vi "wfm_feature calc_repeat_range.vi"(8 "error in (no error)":errorcluster, 10 "limit data":cluster{"X":dbl, "Y":dbl}[](array[cluster]), 11 "wfm_feature in":refnum<class "wfm_feature.lvclass">) -> (0 "error out":errorcluster, 3 "wfm_feature out":refnum<class "wfm_feature.lvclass">)   [LabVIEW 2018, in "wfm_feature.lvclass"]
uses:
  wfm_feature.lvclass
  wfm_feature.lvclass/wfm_feature.ctl
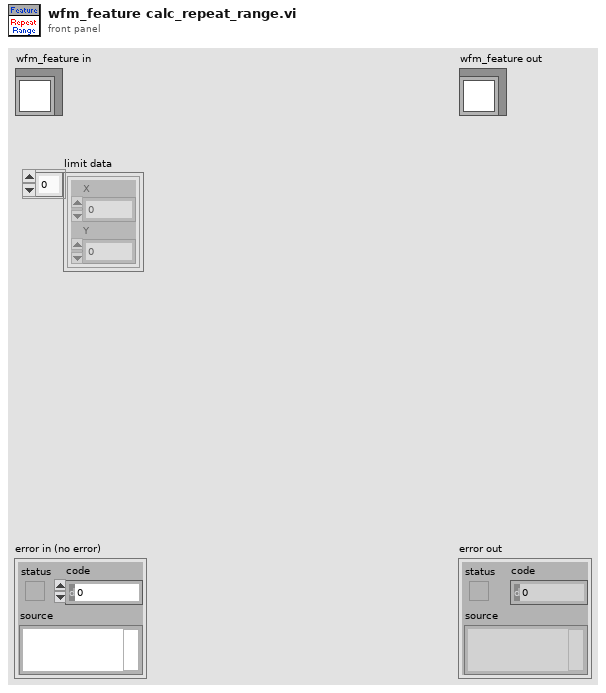
[diagram p1: front panel]
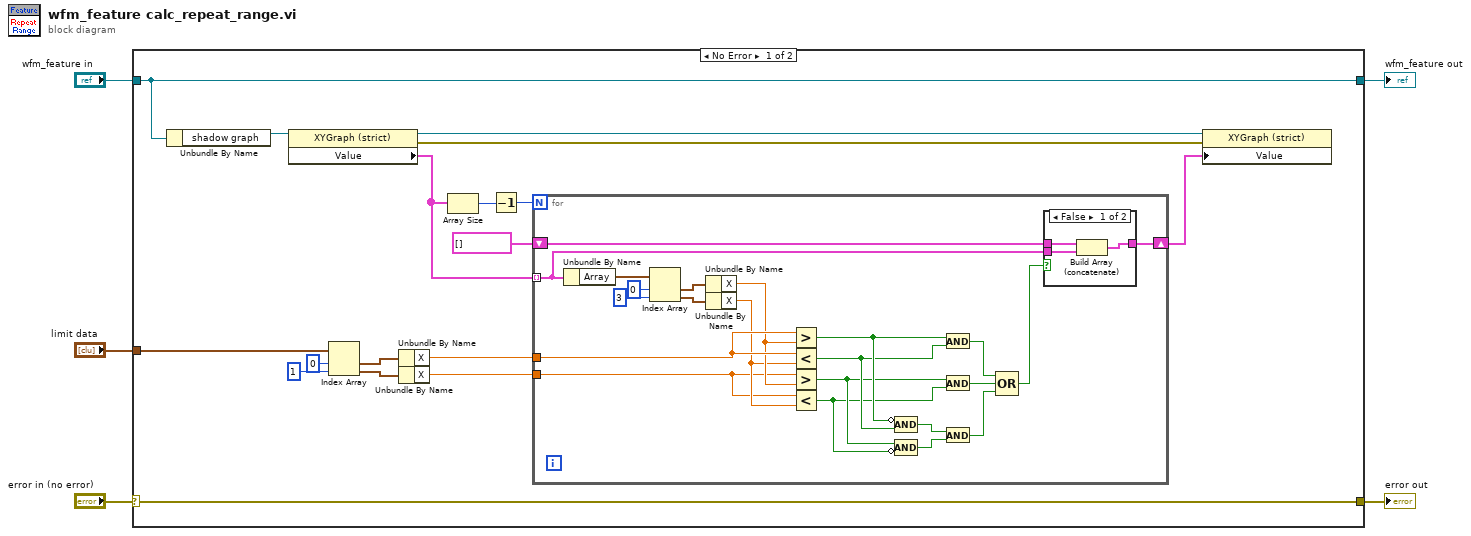
[diagram p0: block diagram]
diagram:
  n1 = case shown="No Error" "error in (no error)" {
    selector: "error in (no error)" -> [w22 w50]
    tunnel: [w22 w50] -> w4
    tunnel: [w6 w49] -> w2
    tunnel: "wfm_feature in" -> [w6 w49]
    tunnel: "limit data" -> [w20 _]
    frame No Error {
      n2 = Unbundle By Name(w6) -> ("shadow graph"=w21:refnum<vi>)
      n3 = property class="XYGraph (strict)"(reference=w21) -> (reference out=w9:refnum<vi>, error out=w8:errorcluster, "Value"=w11:cluster{"Array":cluster{"X":dbl, "Y":dbl}[]}[])  [unwired: 1 in]
      n4 = Index Array(array=w20, index #1=0 ("index"), index #2=1 ("index")) -> (element #1=w17:cluster{"X":dbl, "Y":dbl}, element #2=w16:cluster{"X":dbl, "Y":dbl})
      n5 = Unbundle By Name(w17) -> ("X"=w15:dbl)
      n6 = Unbundle By Name(w16) -> ("X"=w14:dbl)
      n7 = Array Size(array=w11) -> (size(s)=w12:i32)
      n8 = Decrement(x=w12) -> (x-1=w10:i32)
      n9 = for {
        N: w10 -> [_]
        tunnel: w11 -> [w30] mode=indexing
        tunnel: w15 -> [w39]
        tunnel: w14 -> [w36]
        shift-right: [w32] -> w7
        shift-left: cluster{"Array":cluster{"X":dbl, "Y":dbl}[]}[] [] ("Value") -> [w31]
        n10 = Unbundle By Name(w30) -> ("Array"=w44:cluster{"X":dbl, "Y":dbl}[])
        n11 = Index Array(array=w44, index #1=0 ("index"), index #2=3 ("index")) -> (element #1=w41:cluster{"X":dbl, "Y":dbl}, element #2=w40:cluster{"X":dbl, "Y":dbl})
        n12 = Unbundle By Name(w41) -> ("X"=w38:dbl)
        n13 = Unbundle By Name(w40) -> ("X"=w37:dbl)
        n14 = Greater?(x=w39, y=w38) -> (0:w29:bool)
        n15 = Less?(x=w39, y=w37) -> (x < y?=w28:bool)
        n16 = Greater?(x=w36, y=w38) -> (0:w27:bool)
        n17 = Less?(x=w36, y=w37) -> (x < y?=w26:bool)
        n18 = Compound Arithmetic op=AND(invert w29, w28) -> (w25:bool)
        n19 = Compound Arithmetic op=AND(w27, invert w26) -> (w24:bool)
        n20 = And(x=w29, y=w28) -> (x .and. y?=w35:bool)
        n21 = And(x=w27, y=w26) -> (x .and. y?=w34:bool)
        n22 = And(x=w25, y=w24) -> (x .and. y?=w23:bool)
        n23 = Compound Arithmetic op=OR(w35, w34, w23) -> (w33:bool)
        n24 = case shown="False" w33 {
          tunnel: [w45 w48] -> w32
          tunnel: w31 -> [w47 w48]
          tunnel: w30 -> [w46 _]
          frame False {
            n25 = Build Array (concatenate)(w47, w46) -> (w45:cluster{"Array":cluster{"X":dbl, "Y":dbl}[]}[])
          }
          frame True {
          }
        }
      }
      n26 = property class="XYGraph (strict)"(reference=w9, error in=w8, "Value"=w7) -> ()  [unwired: 2 out]
    }
    frame Error {
    }
  }
  "error out" <- w4
  "wfm_feature out" <- w2
